vi "SinExpRootSubVi.vi"(0 "x node":i32, 1 "y node":i32, 2 "time":dbl, 3 "u":dbl, 4 "A":dbl, 5 "w":dbl, 6 "x":dbl, 7 "L":dbl, 9 "k":dbl) -> (14 "SinExpRoot":dbl)   [LabVIEW 2017]
panel:
  out "sqrtPart":dbl
  out "SinPart":dbl
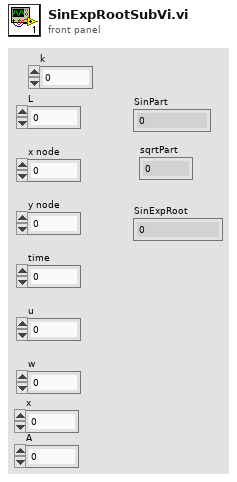
[diagram p1: front panel]
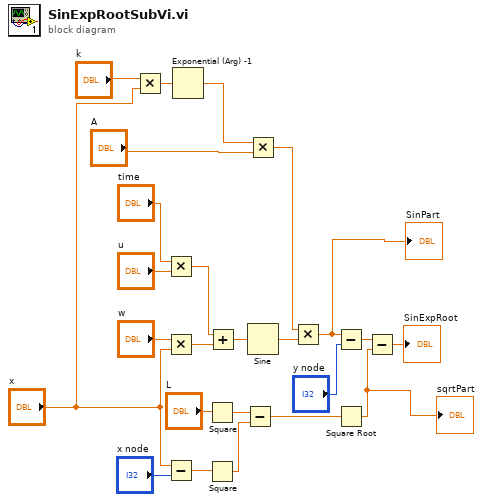
[diagram p0: block diagram]
diagram:
  n1 = Multiply(x="k", y="x") -> (x*y=w4:dbl)
  n2 = Multiply(x="time", y="u") -> (x*y=w18:dbl)
  n3 = Multiply(x="w", y="x") -> (x*y=w17:dbl)
  n4 = Subtract(x="x", y="x node") -> (x-y=w14:dbl)
  n5 = Exponential (Arg) -1(1:w4) -> (0:w3:dbl)
  n6 = Square(x="L") -> (x^2=w10:dbl)
  n7 = Square(x=w14) -> (x^2=w9:dbl)
  n8 = Add(x=w18, y=w17) -> (x+y=w16:dbl)
  n9 = Subtract(x=w10, y=w9) -> (x-y=w11:dbl)
  n10 = Multiply(x=w3, y="A") -> (x*y=w1:dbl)
  n11 = Sine(x=w16) -> (sin(x)=w12:dbl)
  n12 = Multiply(x=w1, y=w12) -> (x*y=w8:dbl)
  "SinPart" <- w8
  n13 = Subtract(x=w8, y="y node") -> (x-y=w15:dbl)
  n14 = Square Root(x=w11) -> (sqrt(x)=w7:dbl)
  "sqrtPart" <- w7
  n15 = Subtract(x=w15, y=w7) -> (x-y=→"SinExpRoot":dbl)
